vi "Create.vi"(8 "error in (no error)":errorcluster) -> (0 "error out":errorcluster, 3 "data value reference":refnum<data-value>)   [LabVIEW 2022 SP3, in "Laser State Data.lvclass"]
uses:
  Laser State Data.lvclass
  Laser State.ctl
  Laser State Data.lvclass/Laser State Data.ctl
  Time and Temp.ctl
panel:
  in  "Time and Temp":T1[](array[typedef])
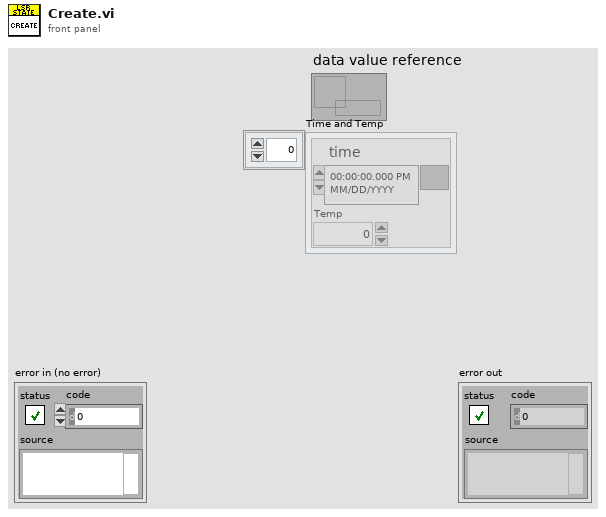
[diagram p1: front panel]
types:
  T1 = typedef "Laser State Data.lvclass/Time and Temp.ctl" = cluster{" time":timestamp, "Temp":dbl}
  T2 = typedef "Laser State Data.lvclass/Laser State.ctl" = enum16{"Idle", "Warming", "Ready", "Firing"}
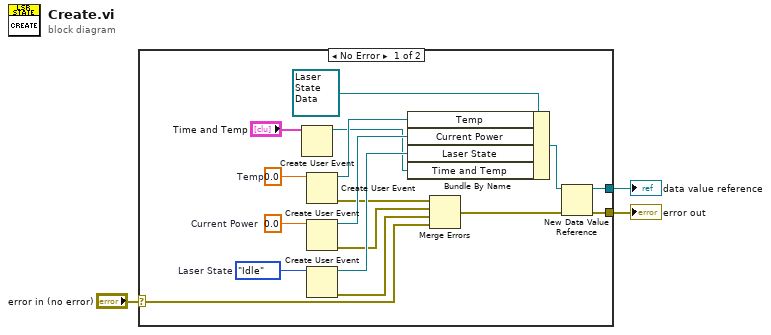
[diagram p0: block diagram]
diagram:
  n1 = case shown="No Error" "error in (no error)" {
    selector: "error in (no error)" -> [w20 w21]
    tunnel: [w7 w21] -> w2
    tunnel: [w6 _] -> w1
    frame No Error {
      w16 = Laser_State."Idle"  # Laser State
      w17 = 0.0  # Current Power
      w18 = 0.0  # Temp
      n2 = Create User Event(user event datatype="Time and Temp") -> (user event=w4:refnum<user-event>)  [unwired: 1 in, 1 out]
      n3 = Create User Event(user event datatype=w18) -> (user event=w15:refnum<user-event>, error out=w12:errorcluster)  [unwired: 1 in]
      n4 = Create User Event(user event datatype=w17) -> (user event=w14:refnum<user-event>, error out=w11:errorcluster)  [unwired: 1 in]
      n5 = Create User Event(user event datatype=w16) -> (user event=w13:refnum<user-event>, error out=w10:errorcluster)  [unwired: 1 in]
      n6 = Bundle By Name(cluster=refnum<class "Laser State Data.lvclass"> refnum ("Laser State Data out"), "Temp"=w15, "Current Power"=w14, "Laser State"=w13, "Time and Temp"=w4) -> (w9:refnum<class "Laser State Data.lvclass">)
      n7 = Merge Errors(w12, w11, w10, w20) -> (w8:errorcluster)
      n8 = New Data Value Reference(data value=w9, error in=w8) -> (data value reference=w6:refnum<data-value>, error out=w7:errorcluster)
    }
    frame Error {
    }
  }
  "error out" <- w2
  "data value reference" <- w1
